vi "Respond.vi"(7 "Publish Data?(F)":bool, 8 "error in (no error)":errorcluster, 9 "Data":refnum<class "Data.lvclass">, 10 "Actor in":refnum<class "Actor.lvclass">, 11 "Response Core in":refnum<class "Interruptible Reply Core.lvclass">) -> (0 "error out":errorcluster, 2 "Actor out":refnum<class "Actor.lvclass">)   [LabVIEW 2020, in "Publisher.lvlib" / "Interruptible Reply Core.lvclass"]
doc: "Handle the Data Action response.\n\nThis implementation enqueues Data on the Reply Queue."
uses:
  Interruptible Reply Core.lvclass
  PPL/HDH.Data.Generic.lvlibp/Data.lvclass
  PPL/HDH.Actor Framework.Core.Actor.lvlibp/1abvi3w/vi.lib/ActorFramework/Actor/Actor.lvclass
  Interruptible Reply Core.lvclass/Interruptible Reply Core.ctl
  PPL/HDH.Data.Generic.lvlibp/Synchronization/Queue/Queue.lvclass
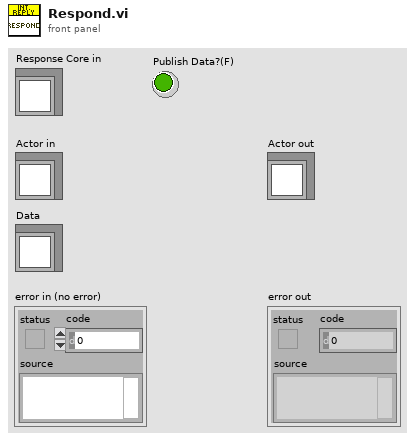
[diagram p1: front panel]
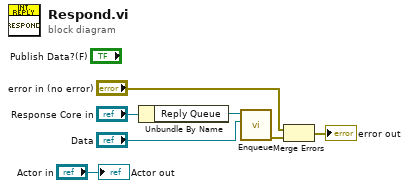
[diagram p0: block diagram]
diagram:
  n1 = Unbundle By Name("Response Core in") -> ("Reply Queue"=w6:refnum<class "Queue.lvclass">)
  n2 = call "Enqueue.vi"("Data to Enqueue"="Data", "Queue in"=w6) -> ("error out"=w3:errorcluster)  [unwired: 7 in, 2 out]
  n3 = Merge Errors("error in (no error)", w3) -> (→"error out":errorcluster)
  "Actor out" <- "Actor in"
